vi "chart set series overlap.vi"(8 "error in (no error)":errorcluster, 10 "overlap":i8, 11 "chart":u32) -> (0 "error out":errorcluster)   [LabVIEW 2015, in "xlsxwriter.lvlib"]
doc: "void chart_set_series_overlap(lxw_chart chart, int8_t overlap);"
uses:
  xlsxwriter.lvlib
  xlsxwriter.dll
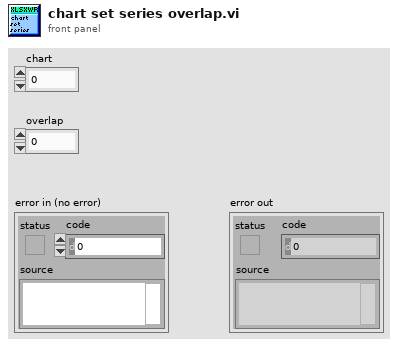
[diagram p1: front panel]
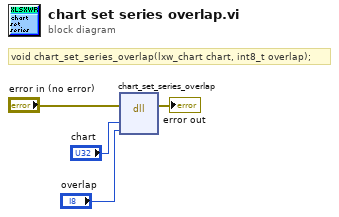
[diagram p0: block diagram]
diagram:
  # "void chart_set_series_overlap(lxw_chart chart, int8_t overlap);"
  n1 = dll-call lib="C:/Users/WDAGUtilityAccount/Desktop/lv_vis_added_cell/xlsxwriter.*" fn="chart_set_series_overlap"(error in="error in (no error)", "chart"="chart", "overlap"="overlap") -> (error out=→"error out":errorcluster)  [unwired: 5 in, 1 out]
